vi "CLFN.vi"   [LabVIEW 2013, in "NISE Tools Drop Templates.lvlib"]
uses:
  NISE Tools Drop Templates.lvlib
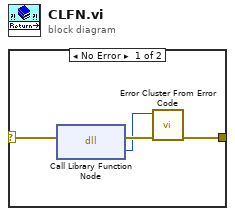
[diagram p0: block diagram]
diagram:
  n1 = case shown="No Error" {
    selector: _ -> [w2 w5]
    tunnel: [w1 w5] -> _
    frame No Error {
      n2 = dll-call lib="?" fn="Call Library Function Node"(error in=w2) -> (error out=w4:errorcluster, "return type"=w3:i32)  [unwired: 2 in, 1 out]
      n3 = call <vilib>:"Error Cluster From Error Code.vi"("error in (no error)"=w4, "error code (0)"=w3) -> ("error out"=w1:errorcluster)  [unwired: 7 in]
    }
    frame Error {
    }
  }
